vi "task_2.vi"() -> ()   [LabVIEW 2023]
panel:
  out "Output":u64
  in  "stop":bool
  in  "Options":T1(ring)
  in  "Input N":i32
  in  "Input M":i32
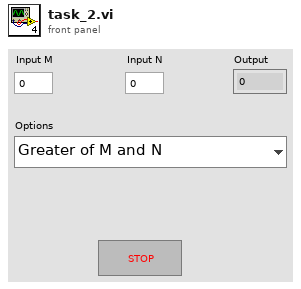
[diagram p1: front panel]
types:
  T1 = enum16{"Greater of M and N ", "Sum of factorials of first N whole numbers ", "Sum of factorials of first M natural numbers ", "Factorial of M+N "}
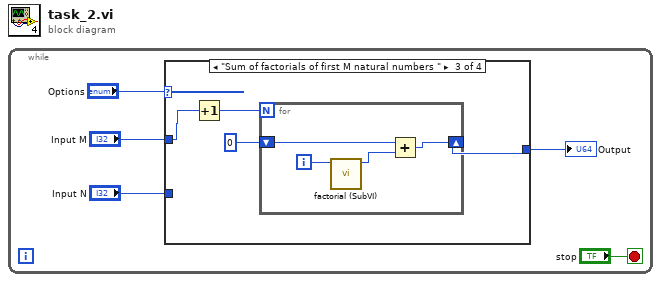
[diagram p0: block diagram]
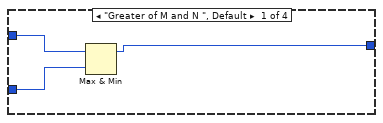
[diagram p2: hidden frame]
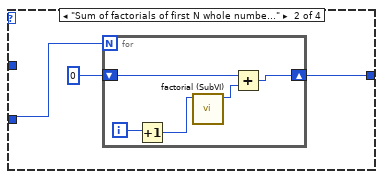
[diagram p3: hidden frame]
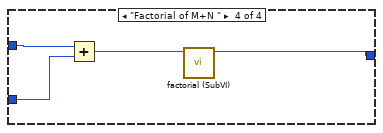
[diagram p4: hidden frame]
diagram:
  n1 = while {
    stop <- "stop" stop-if-true
    n2 = case shown="\"Sum of factorials of first M natural numbers \"" "Options" {
      tunnel: "Input M" -> [w8 _ w17 w28]
      tunnel: "Input N" -> [w7 w11 _ w27]
      tunnel: [w6 w9 w19 w25] -> w1
      frame "Greater of M and N ", Default {
        n3 = Max & Min(x=w8, y=w7) -> (max(x,y)=w6:i32)  [unwired: 1 out]
      }
      frame "Sum of factorials of first N whole numbers " {
        n4 = for {
          N: w11 -> [_]
          shift-right: [w12] -> w9
          shift-left: u64 0 -> [w16]
          i -> [w14]
          n5 = Increment(x=w14) -> (x+1=w13:i32)
          n6 = call "factorial (SubVI).vi"("Num"=w13) -> ("Numeric"=w15:u64)  [unwired: 10 in]
          n7 = Add(x=w16, y=w15) -> (x+y=w12:u64)
        }
      }
      frame "Sum of factorials of first M natural numbers " {
        n8 = Increment(x=w17) -> (x+1=w18:i32)
        n9 = for {
          N: w18 -> [_]
          shift-right: [w23] -> w19
          shift-left: u64 0 -> [w24]
          i -> [w22]
          n10 = call "factorial (SubVI).vi"("Num"=w22) -> ("Numeric"=w21:u64)  [unwired: 10 in]
          n11 = Add(x=w24, y=w21) -> (x+y=w23:u64)
        }
      }
      frame "Factorial of M+N " {
        n12 = Add(x=w28, y=w27) -> (x+y=w26:i32)
        n13 = call "factorial (SubVI).vi"("Num"=w26) -> ("Numeric"=w25:u64)  [unwired: 10 in]
      }
    }
    "Output" <- w1
  }
